vi "Test03_PIPELINE.vi"() -> ()   [LabVIEW 2018]
uses:
  <userlib>/_MGI/1D Array/MGI Average/MGI Average (DBL[]).vi
panel:
  in  "Close Radio (in)":i32=1
  in  "Open Radio (in)":i32=1
  in  "Dilate Radio (in)":i32=1
  out "Close Time (ms)":dbl
  out "Open Time (ms)":dbl
  out "Dilate Time (ms)":dbl
  in  "Erode Radio (in)":i32=1
  out "Erode Time (ms)":dbl
  out "Mean Time (ms)":dbl
  out "Elapsed Time (s)":dbl
  out "Image Out":T1(plugin-control)
  out "Image In":T1(plugin-control)
  out "Error Out":errorcluster
  in  "Error In":errorcluster
  out "Processed Images":i32
  in  "Start":bool
  out "error_cuda_free":i32
  out "error_gpu_to_cpu":i32
  out "error_cpu_to_gpu":i32
  out "Cuda Free (ms)":dbl
  out "Set IMG Param (ms)":dbl
  out "Total (ms)":dbl
  out "Copy to CPU (ms)":dbl
  out "Threshold (ms)":dbl
  out "Copy to GPU (ms)":dbl
  in  "Stop":bool
  in  "max":i32=240
  in  "min":i32=70
  in  "Folder Path":path=path "C:/Users/AUTIS/Documents/TFG/Proyecto/Imagenes"
  # "GPU CUDA -"
  # "PIPELINE"
  # "Configuration"
  # "Threshold Parameters"
  # "Erode Parameters"
  # "Dilate Parameters"
  # "Time Results"
  # "General Info"
  # "Errors Info"
  # "Open Parameters"
  # "Close Parameters"
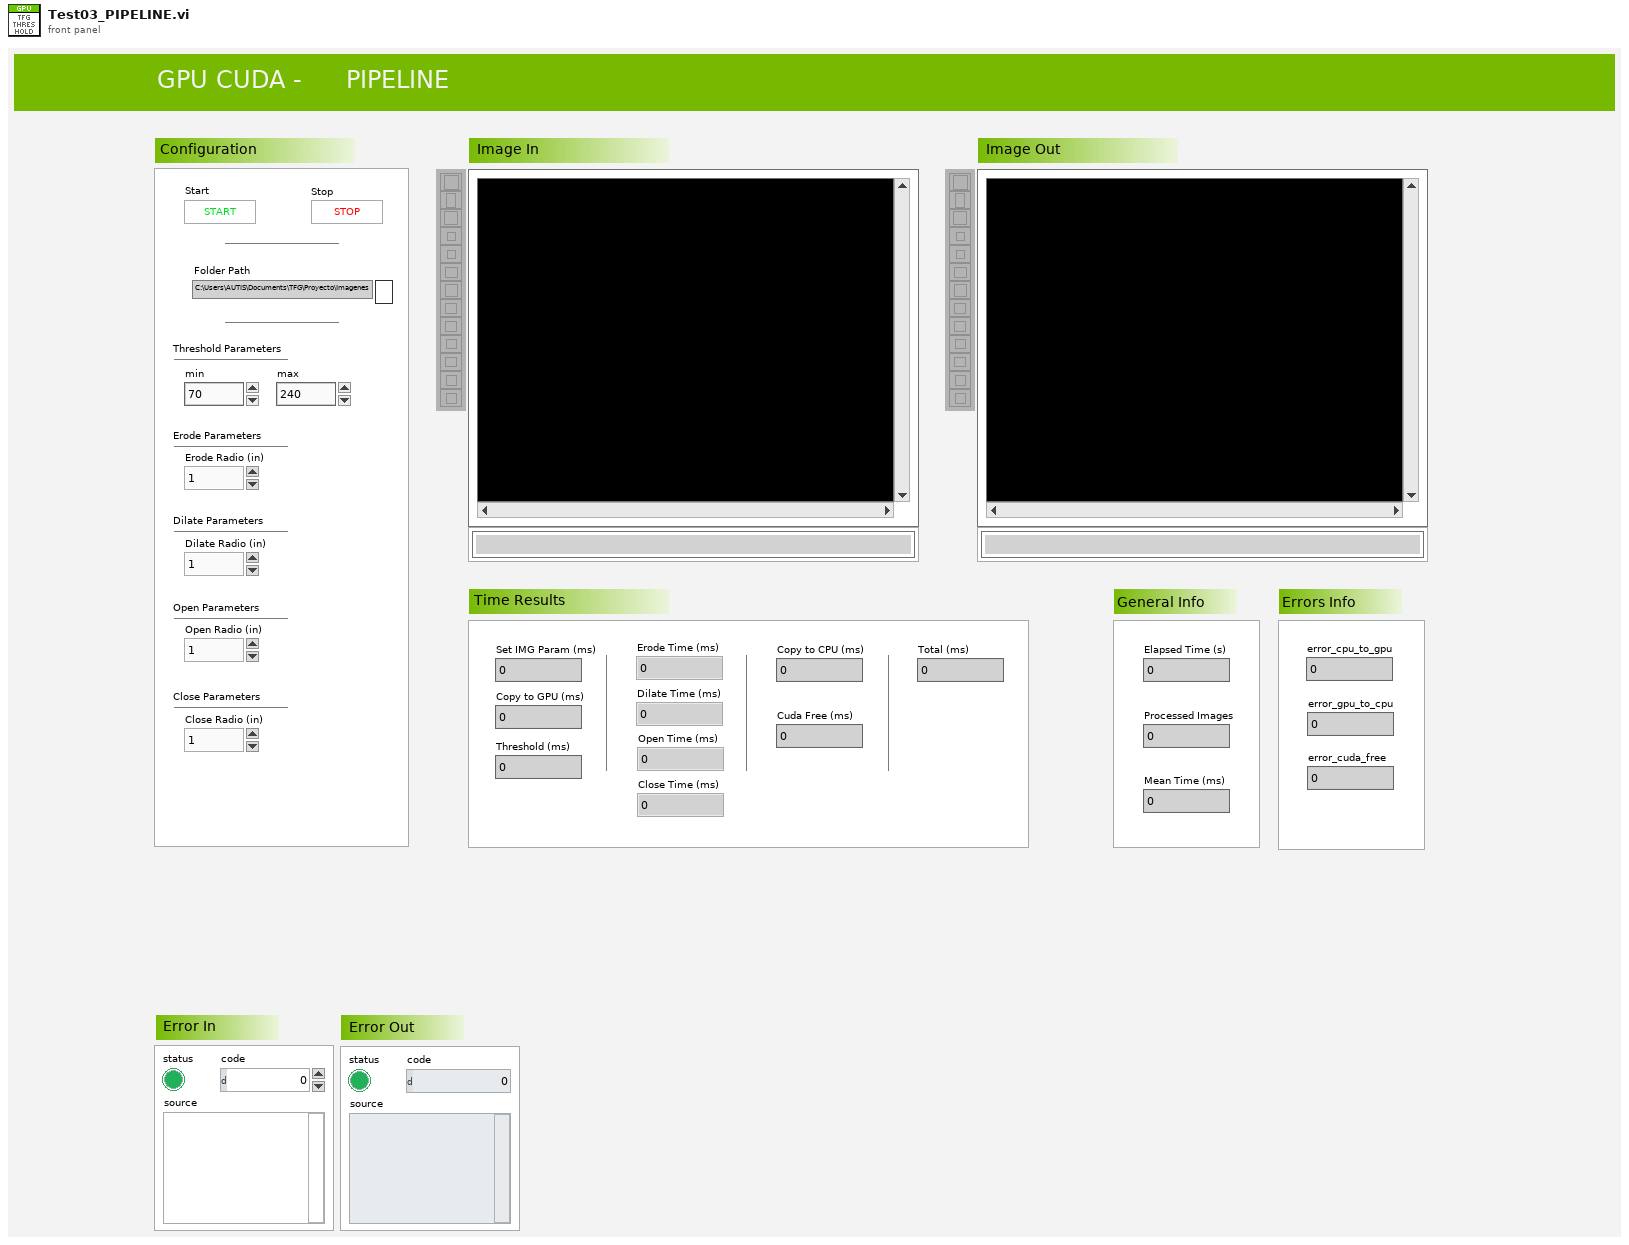
[diagram p1: front panel]
types:
  T1 = typedef "IMAQ Image.ctl" = refnum<image>
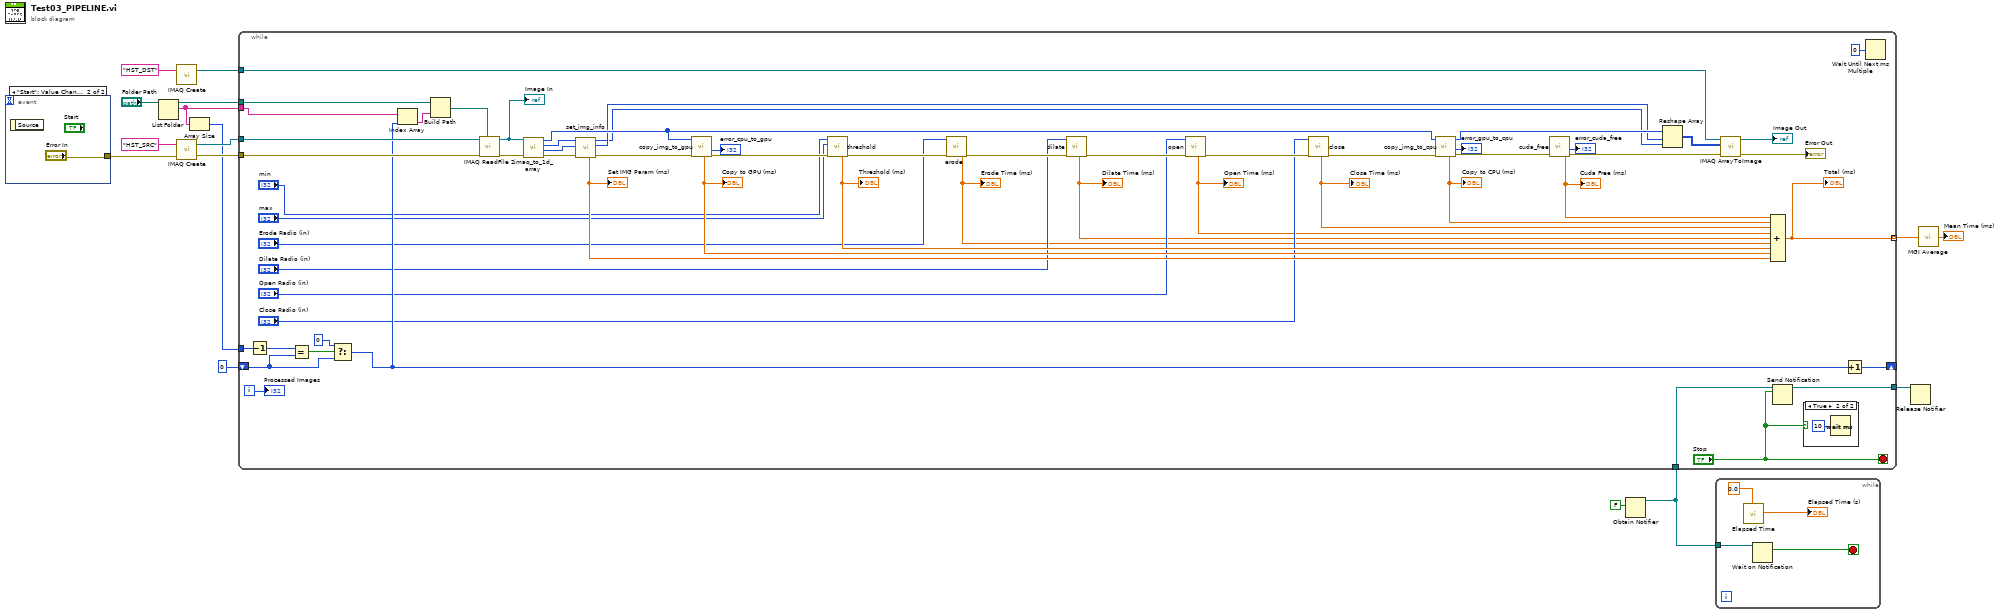
[diagram p0: block diagram]
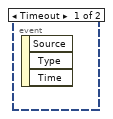
[diagram p2: hidden frame]
diagram:
  n1 = event shown="[1] \"Start\": Value Change" {
    selector: _ -> [_ _]
    dyn-events: _ -> [_ _]
    timeout: _ -> [_ _]
    tunnel: [_ "Error In"] -> w6
    event Timeout {
      n2 = event-data() -> ()  [unwired: 1 in, 3 out]
    }
    event "Start": Value Change {
      n3 = event-data() -> ()  [unwired: 1 in, 1 out]
    }
  }
  n4 = List Folder(path="Folder Path") -> (path out=w10:path, filenames=w9:string[])  [unwired: 3 in, 2 out]
  n5 = call "IMAQ Create"("Image Name"="HST_DST") -> ("New Image"=w13:T1)  [unwired: 4 in, 1 out]
  n6 = call "IMAQ Create"("Image Name"="HST_SRC", "error in (no error)"=w6) -> ("New Image"=w15:T1, "error out"=w12:errorcluster)  [unwired: 3 in]
  n7 = Array Size(array=w9) -> (size(s)=w8:i32)
  n8 = Obtain Notifier(notification data type=FALSE) -> (notifier out=w3:refnum<notifier>)  [unwired: 3 in, 2 out]
  n9 = while {
    tunnel: w15 -> [w76]
    tunnel: w10 -> [w52]
    tunnel: w13 -> [w75]
    tunnel: w12 -> [w72]
    tunnel: w9 -> [w50]
    tunnel: w8 -> [w47]
    shift-right: [w45] -> _
    shift-left: 0 -> [w41]
    tunnel: w3 -> [w35]
    tunnel: [w34] -> w4
    tunnel: [w33] -> w2 mode=indexing
    i -> [w48]
    stop <- "Stop" stop-if-true
    n10 = Decrement(x=w47) -> (x-1=w46:i32)
    n11 = Equal?(x=w46, y=w41) -> (x = y?=w44:bool)
    n12 = Select(t=0, s=w44, f=w41) -> (s? t:f=w42:i32)
    n13 = Index Array(array=w50, index=w42) -> (element=w49:string)
    n14 = Build Path(base path=w52, name or relative path=w49) -> (appended path=w51:path)
    n15 = call "IMAQ ReadFile 2"("File Path"=w51, "error in (no error)"=w72, "Image"=w76) -> ("error out"=w59:errorcluster, "Image Out"=w39:T1)  [unwired: 4 in, 3 out]
    "Image In" <- w39
    n16 = call "imaq_to_1d_array.vi"("Error in"=w59, "Image (in)"=w39) -> ("Error out"=w58:errorcluster, "Height"=w55:i32, "Width"=w56:i32, "Hst Src Image array (out)"=w57:u8[])  [unwired: 6 in]
    n17 = call "set_img_info.vi"("Error in"=w58, "Height (in)"=w55, "Width (in)"=w56) -> ("Error out"=w69:errorcluster, "Height (out)"=w54:i32, "Width (out)"=w53:i32, "Set IMG Parameters Time (ms)"=w68:dbl)  [unwired: 5 in]
    "Set IMG Param (ms)" <- w68
    n18 = call "copy_img_to_gpu.vi"("Error in"=w69, "Hst Src Image (in)"=w57) -> ("Error out"=w60:errorcluster, "error_code"=→"error_cpu_to_gpu":i32, "Copy to GPU Time (ms)"=w70:dbl)  [unwired: 6 in, 1 out]
    "Copy to GPU (ms)" <- w70
    n19 = call "threshold.vi"("Error in"=w60, "Threshold max (in)"="max", "Threshold min (in)"="min") -> ("Error out"=w31:errorcluster, "Threshold Time (ms)"=w61:dbl)  [unwired: 4 in, 3 out]
    "Threshold (ms)" <- w61
    n20 = call "erode.vi"("Error in"=w31, "Erode Radio (in)"="Erode Radio (in)") -> ("Error out"=w28:errorcluster, "Erode Time (ms)"=w18:dbl)  [unwired: 6 in, 2 out]
    "Erode Time (ms)" <- w18
    n21 = call "dilate.vi"("Error in"=w28, "Dilate Radio (in)"="Dilate Radio (in)") -> ("Error out"=w27:errorcluster, "Dilate Time (ms)"=w19:dbl)  [unwired: 6 in, 2 out]
    "Dilate Time (ms)" <- w19
    n22 = call "open.vi"("Error in"=w27, "Open Radio (in)"="Open Radio (in)") -> ("Error out"=w26:errorcluster, "Open Time (ms)"=w20:dbl)  [unwired: 6 in, 2 out]
    "Open Time (ms)" <- w20
    n23 = call "close.vi"("Error in"=w26, "Close Radio (in)"="Close Radio (in)") -> ("Error out"=w25:errorcluster, "Close Time (ms)"=w21:dbl)  [unwired: 6 in, 2 out]
    "Close Time (ms)" <- w21
    n24 = call "copy_img_to_cpu.vi"("Error in"=w25, "Hst Dst Image (in)"=w57) -> ("Error out"=w67:errorcluster, "error_code"=→"error_gpu_to_cpu":i32, "Hst Dst Image (out)"=w74:u8[], "Copy to CPU Time (ms)"=w73:dbl)  [unwired: 6 in]
    "Copy to CPU (ms)" <- w73
    n25 = call "cuda_free.vi"("Error in"=w67) -> ("Error out"=w66:errorcluster, "error_code"=→"error_cuda_free":i32, "Cuda Free Time (ms)"=w65:dbl)  [unwired: 8 in]
    "Cuda Free (ms)" <- w65
    n26 = Reshape Array(w74, w54, w53) -> (w71:u8[][])
    n27 = call "IMAQ ArrayToImage"("error in (no error)"=w66, "Image Pixels (U8)"=w71, "Image"=w75) -> ("error out"=→"Error Out":errorcluster, "Image Out"=→"Image Out":T1)  [unwired: 7 in]
    n28 = Compound Arithmetic op=ADD(w65, w73, w21, w20, w19, w18, w61, w70, w68) -> (w33:dbl)
    "Total (ms)" <- w33
    n29 = Send Notification(notification="Stop", notifier=w35) -> (notifier out=w34:refnum<notifier>)  [unwired: 1 in, 1 out]
    n30 = case shown="True" "Stop" {
      frame False {
      }
      frame True {
        n31 = Wait (ms)(milliseconds to wait=u32 10) -> ()  [unwired: 1 out]
      }
    }
    n32 = Increment(x=w42) -> (x+1=w45:i32)
    n33 = Wait Until Next ms Multiple(millisecond multiple=u32 0) -> ()  [unwired: 1 out]
    "Processed Images" <- w48
  }
  n34 = while {
    tunnel: w3 -> [w81]
    stop <- w79 stop-if-true
    n35 = call "Elapsed Time"("Set Start Time (s)"=0.0) -> ("Elapsed Time (s)"=→"Elapsed Time (s)":dbl)  [unwired: 11 in, 7 out]
    n36 = Wait on Notification(notifier=w81) -> (notification=w79:bool)  [unwired: 3 in, 3 out]
  }
  n37 = Release Notifier(notifier=w4) -> ()  [unwired: 2 in, 3 out]
  n38 = call-poly <userlib>:"MGI Average.vi"("Double[]"=w2) -> ("Average"=→"Mean Time (ms)":dbl)  [unwired: 1 in]
